vi "Check experiment header type.vi"(8 "error in (no error)":errorcluster, 10 "Experiment Header string":refnum<vi>, 11 "Path":path) -> (0 "error out":errorcluster, 2 "Old format ?":bool, 3 "Path- out":path)   [LabVIEW 2017]
uses:
  <vilib>/Utility/config.llb/NI_LVConfig.lvlib
panel:
  out "section names":string[](array[string])
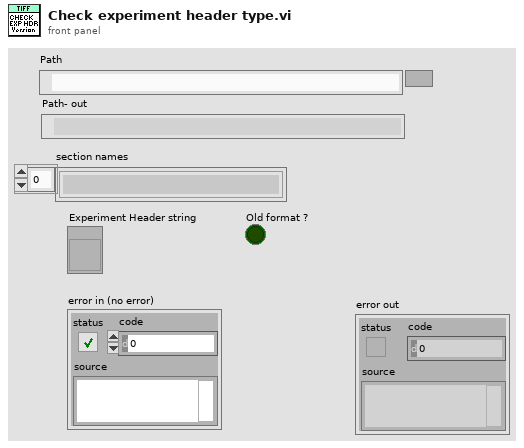
[diagram p1: front panel]
types:
  T1 = typedef "NI_LVConfig.lvlib/Config Data RefNum.ctl" = refnum<k1>
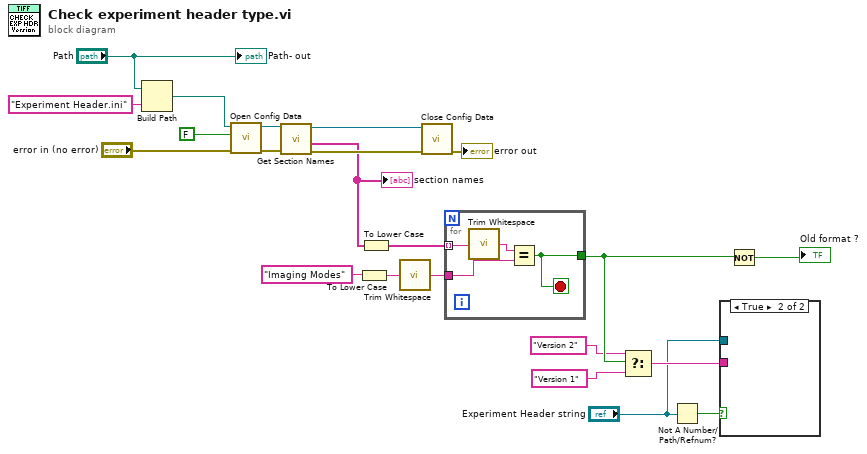
[diagram p0: block diagram]
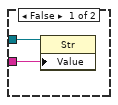
[diagram p2: hidden frame]
diagram:
  n1 = Build Path(base path="Path", name or relative path="Experiment Header.ini") -> (appended path=w20:path)
  n2 = call <vilib>:"Open Config Data.vi"("error in (no error)"="error in (no error)", "create file if necessary (T)"=FALSE, "configuration file path"=w20) -> ("error out"=w17:errorcluster, "refnum"=w16:T1)  [unwired: 6 in, 1 out]
  n3 = call <vilib>:"Get Section Names.vi"("error in (no error)"=w17, "refnum"=w16) -> ("error out"=w15:errorcluster, "section names"=w12:string[], "refnum out"=w14:T1)  [unwired: 7 in]
  "section names" <- w12
  n4 = To Lower Case(string="Imaging Modes") -> (all lower case string=w10:string)
  n5 = To Lower Case(string=w12) -> (all lower case string=w8:string[])
  n6 = call <vilib>:"Trim Whitespace.vi"("string"=w10) -> ("trimmed string"=w9:string)  [unwired: 1 in]
  n7 = call <vilib>:"Close Config Data.vi"("error in (no error)"=w15, "refnum"=w14) -> ("error out"=→"error out":errorcluster)  [unwired: 8 in, 1 out]
  n8 = for {
    tunnel: w9 -> [w26]
    tunnel: w8 -> [w25] mode=indexing
    tunnel: [w23] -> w6
    stop <- w23 stop-if-true
    n9 = call <vilib>:"Trim Whitespace.vi"("string"=w25) -> ("trimmed string"=w24:string)  [unwired: 1 in]
    n10 = Equal?(x=w24, y=w26) -> (x = y?=w23:bool)
  }
  n11 = Select(t="Version 2", s=w6, f="Version 1") -> (s? t:f=w2:string)
  n12 = Not A Number/Path/Refnum?(number/path/refnum="Experiment Header string") -> (NaN/Path/Refnum?=w3:bool)
  n13 = case shown="True" w3 {
    tunnel: w2 -> [w28 _]
    tunnel: "Experiment Header string" -> [w27 _]
    frame False {
      n14 = property class="Str"(reference=w27, "Value"=w28) -> ()  [unwired: 1 in, 2 out]
    }
    frame True {
    }
  }
  n15 = Not(x=w6) -> (.not. x?=→"Old format ?":bool)
  "Path- out" <- "Path"
